vi "Read from XML File and Unflatten Data.vi"() -> ()   [LabVIEW 2023]
doc: "Reads an array of data, including the max, min, and average values from an XML file created by the Flatten Data and Write to XML File.vi example. The VI then unflattens this data to LabVIEW data and displays it on the front panel."
uses:
  support/Random Graph Data.ctl
  <vilib>/Utility/xml.llb/Read From XML File(string).vi
  <vilib>/Utility/xml.llb/Read From XML File(array).vi
panel:
  out "Retrieved XML":string
  out "Graph":T1(graph)
  out "Max":dbl
  out "Min":dbl
  out "Mean":dbl
  # "Overview: Demonstrates the use of the LabVIEW Schema VIs and functions to read data from an XML file (that follows the LabVIEW-specific schema) and unflatten it.\nInstructions:\n1. Make sure you have already run Flatten Data and Write to XML File.vi.\n2. Run this VI. The contents of the XML file will be displayed below.\n3. Delete the XML file (located at [LabVIEW Data]\\Example Flattened XML File.xml) when you are done."
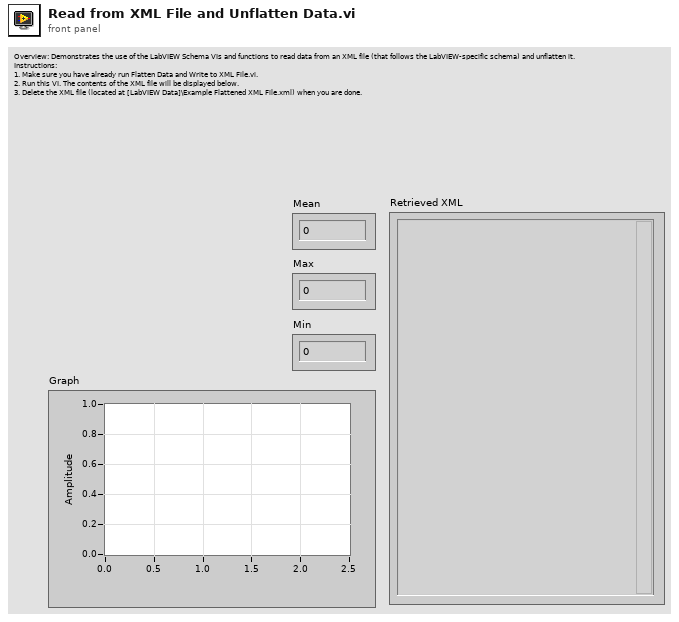
[diagram p1: front panel]
types:
  T1 = cluster{"Initial X":dbl, "Delta X":dbl, "Values":dbl[]}
  T2 = typedef "Random Graph Data.ctl" = cluster{"Initial X":dbl, "Delta X":dbl, "Values":dbl[]}
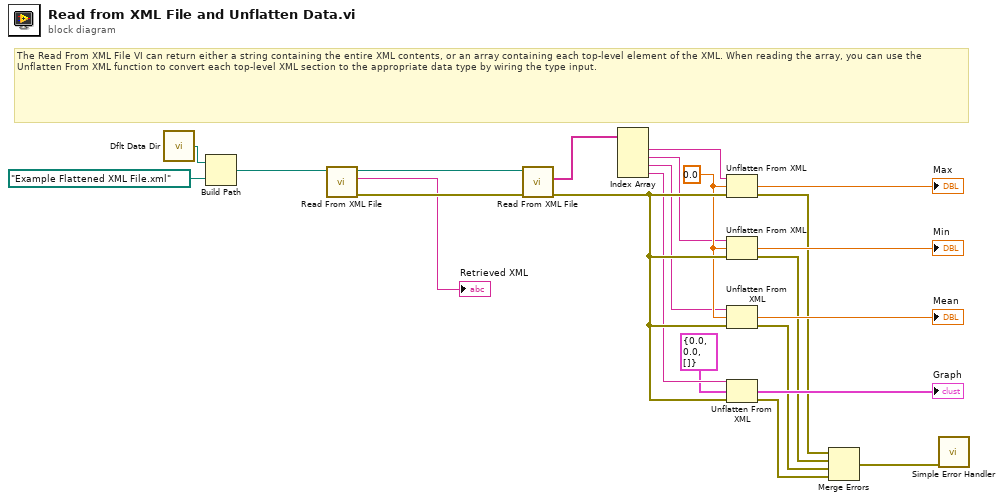
[diagram p0: block diagram]
diagram:
  w17 = 0.0 ("Mean")
  # "The Read From XML File VI can return either a string containing the entire XML contents, or an array containing each top-level element of the XML. When reading the array, you can use the Unflatten From XML function to convert each top-level XML section to the appropriate data type by wiring the type input."
  n1 = call <vilib>:"Dflt Data Dir.vi"() -> ("App:Default Data Directory"=w4:path)
  n2 = Build Path(base path=w4, name or relative path=path "Example Flattened XML File.xml" ("default name")) -> (appended path=w2:path)
  n3 = call-poly <vilib>:"Read From XML File.vi"("XML File Path"=w2) -> ("error out"=w6:errorcluster, "XML Elements"=→"Retrieved XML":string, "XML File Path(duplicate)"=w7:path)  [unwired: 8 in]
  n4 = call-poly <vilib>:"Read From XML File.vi"("error in (no error)"=w6, "XML File Path"=w7) -> ("error out"=w21:errorcluster, "XML Elements"=w23:string[])  [unwired: 7 in, 1 out]
  n5 = Index Array(array=w23) -> (element #1=w16:string, element #2=w11:string, element #3=w10:string, element #4=w9:string)  [unwired: 4 in]
  n6 = Unflatten From XML(xml string=w16, type=w17, error in (no error)=w21) -> (value=→"Max":dbl, error out=w15:errorcluster)
  n7 = Unflatten From XML(xml string=w11, type=w17, error in (no error)=w21) -> (value=→"Min":dbl, error out=w14:errorcluster)
  n8 = Unflatten From XML(xml string=w10, type=w17, error in (no error)=w21) -> (value=→"Mean":dbl, error out=w13:errorcluster)
  n9 = Unflatten From XML(xml string=w9, type=T2 {"Initial X"=0.0, "Delta X"=0.0, "Values"=[]} ("Random Graph Data"), error in (no error)=w21) -> (value=→"Graph":T2, error out=w12:errorcluster)
  n10 = Merge Errors(w15, w14, w13, w12) -> (w3:errorcluster)
  n11 = call <vilib>:"Simple Error Handler.vi"("error in (no error)"=w3) -> ()  [unwired: 4 in, 5 out]
